vi "四点权值_黑子.vi"(0 "3位置行":dbl, 1 "2位置行":dbl, 2 "1位置行":dbl, 3 "当前棋盘状态":i32[][](array[numeric]), 5 "4位置行":dbl, 9 "1位置列":u8, 11 "2位置列":u8, 12 "3位置列":u8, 13 "4位置列":u8) -> (4 "黑子四位置权值":i32, 6 "有2个黑子?或黑子加无子?":bool, 8 "第1个位置是黑子?":bool, 10 "3个黑子?":bool, 14 "第一个位置为空":bool, 15 "3个黑子？或2个黑子加无子?":bool)   [LabVIEW 2018]
doc: "计算当前位置周围4个点的权值。"
panel:
  out "第四位在框内？":bool
  out "第三位在框内？":bool
  out "第二位在框内？":bool
  out "第一位在框内？":bool
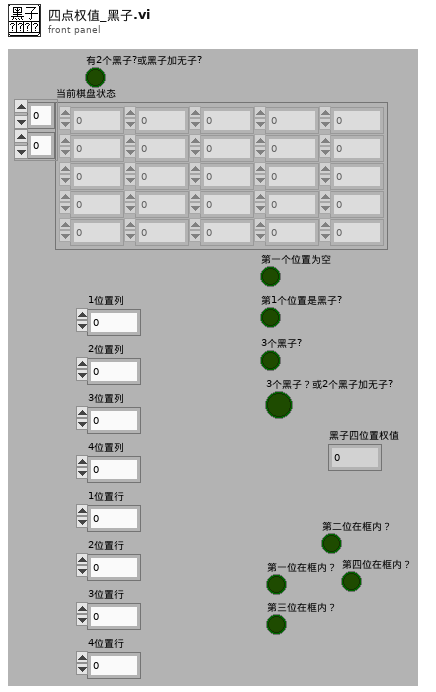
[diagram p1: front panel]
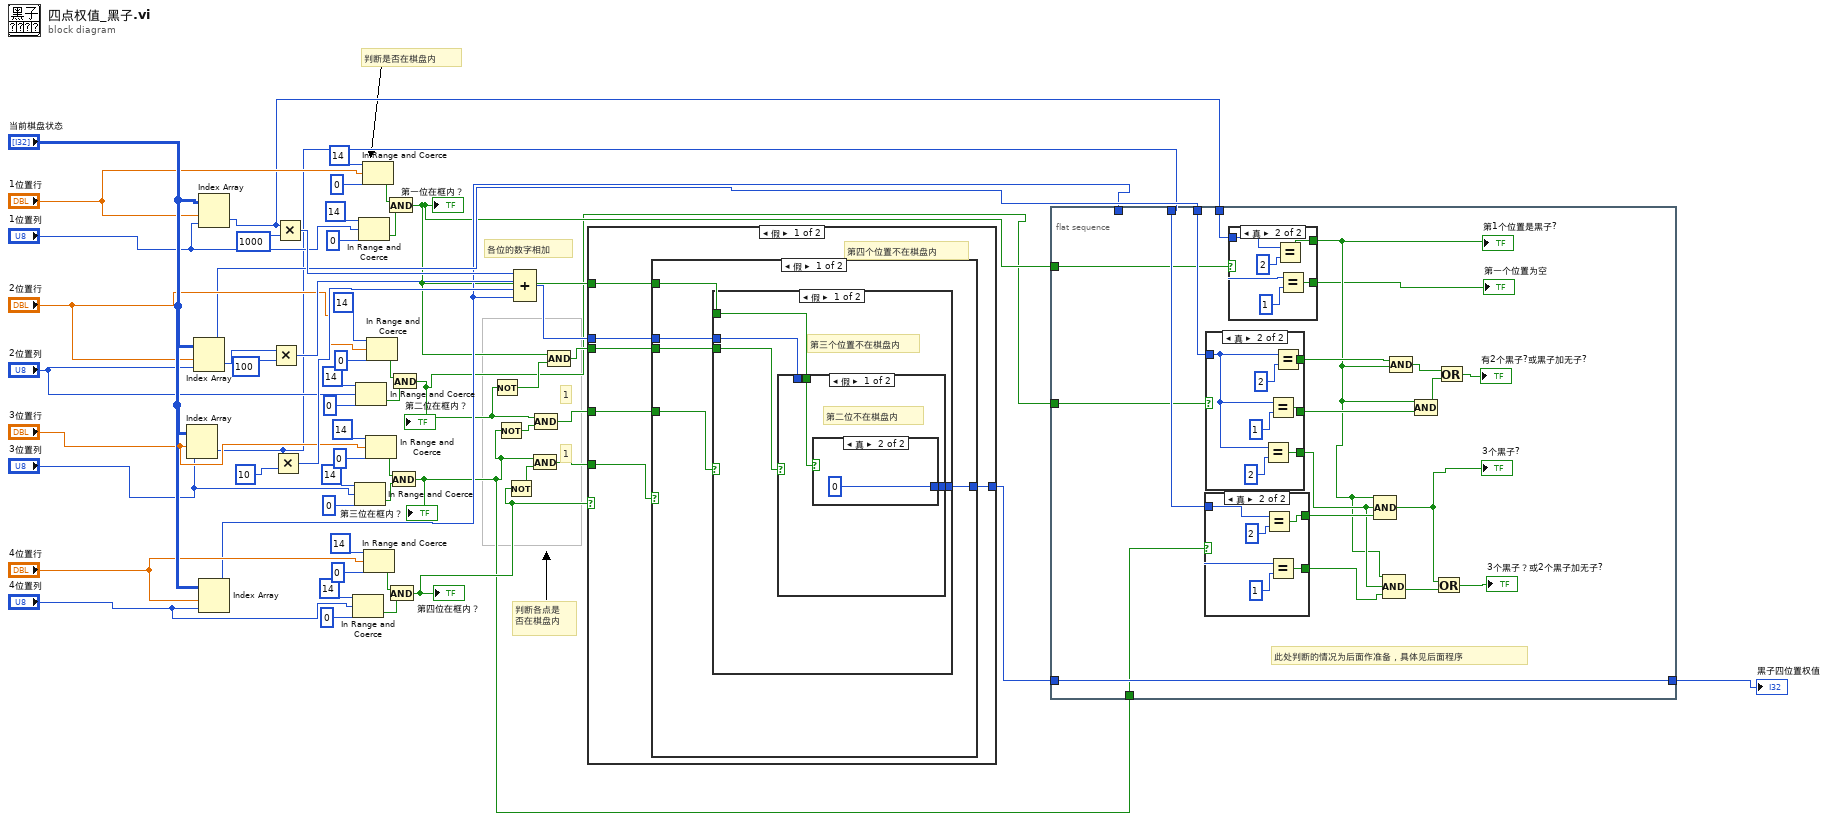
[diagram p0: block diagram]
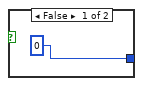
[diagram p2: hidden frame]
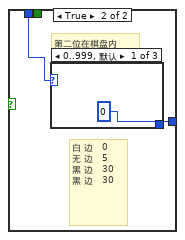
[diagram p3: hidden frame]
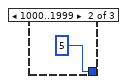
[diagram p4: hidden frame]
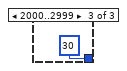
[diagram p5: hidden frame]
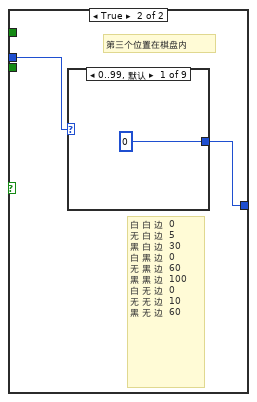
[diagram p6: hidden frame]
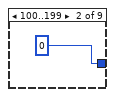
[diagram p7: hidden frame]
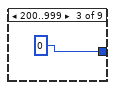
[diagram p8: hidden frame]
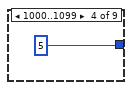
[diagram p9: hidden frame]
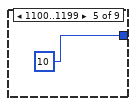
[diagram p10: hidden frame]
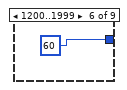
[diagram p11: hidden frame]
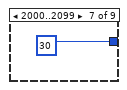
[diagram p12: hidden frame]
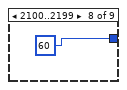
[diagram p13: hidden frame]
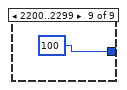
[diagram p14: hidden frame]
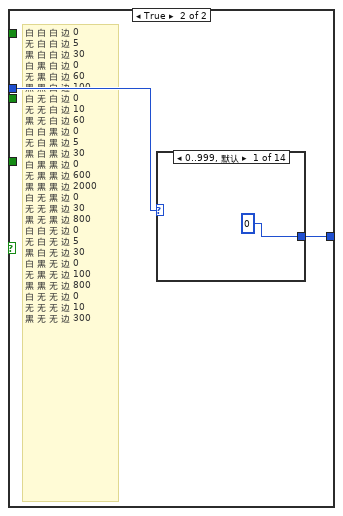
[diagram p15: hidden frame]
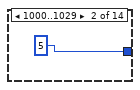
[diagram p16: hidden frame]
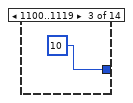
[diagram p17: hidden frame]
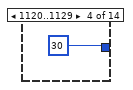
[diagram p18: hidden frame]
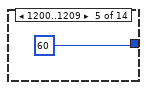
[diagram p19: hidden frame]
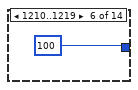
[diagram p20: hidden frame]
diagram:
  # "判断各点是\n否在棋盘内"
  # "各位的数字相加"
  # "判断是否在棋盘内"
  # "1"
  # "1"
  n1 = Index Array(array="当前棋盘状态", index (row)="3位置行", index (col)="3位置列") -> (element=w5:i32)
  n2 = Index Array(array="当前棋盘状态", index (row)="2位置行", index (col)="2位置列") -> (element=w6:i32)
  n3 = Index Array(array="当前棋盘状态", index (row)="1位置行", index (col)="1位置列") -> (element=w7:i32)
  n4 = Index Array(array="当前棋盘状态", index (row)="4位置行", index (col)="4位置列") -> (element=w4:i32)
  n5 = Multiply(x=w6, y=100) -> (x*y=w21:i32)
  n6 = Multiply(x=w5, y=10) -> (x*y=w20:i32)
  n7 = Multiply(x=w7, y=1000) -> (x*y=w22:i32)
  n8 = In Range and Coerce(upper limit=14, x="4位置列", lower limit=0) -> (In Range?=w36:bool)  [unwired: 1 out]
  n9 = In Range and Coerce(upper limit=14, x="3位置列", lower limit=0) -> (In Range?=w30:bool)  [unwired: 1 out]
  n10 = In Range and Coerce(upper limit=14, x="2位置列", lower limit=0) -> (In Range?=w50:bool)  [unwired: 1 out]
  n11 = In Range and Coerce(upper limit=14, x="1位置列", lower limit=0) -> (In Range?=w51:bool)  [unwired: 1 out]
  n12 = In Range and Coerce(upper limit=14, x="1位置行", lower limit=0) -> (In Range?=w52:bool)  [unwired: 1 out]
  n13 = In Range and Coerce(upper limit=14, x="4位置行", lower limit=0) -> (In Range?=w37:bool)  [unwired: 1 out]
  n14 = In Range and Coerce(upper limit=14, x="3位置行", lower limit=0) -> (In Range?=w31:bool)  [unwired: 1 out]
  n15 = In Range and Coerce(upper limit=14, x="2位置行", lower limit=0) -> (In Range?=w49:bool)  [unwired: 1 out]
  n16 = And(x=w52, y=w51) -> (x .and. y?=w3:bool)
  "第一位在框内？" <- w3
  n17 = And(x=w37, y=w36) -> (x .and. y?=w28:bool)
  "第四位在框内？" <- w28
  n18 = And(x=w31, y=w30) -> (x .and. y?=w1:bool)
  "第三位在框内？" <- w1
  n19 = And(x=w49, y=w50) -> (x .and. y?=w2:bool)
  "第二位在框内？" <- w2
  n20 = Not(x=w2) -> (.not. x?=w26:bool)
  n21 = Not(x=w1) -> (.not. x?=w24:bool)
  n22 = Not(x=w28) -> (.not. x?=w25:bool)
  n23 = Compound Arithmetic op=ADD(w22, w21, w20, w4) -> (w19:i32)
  n24 = And(x=w1, y=w25) -> (x .and. y?=w29:bool)
  n25 = Compound Arithmetic op=AND(w2, w24) -> (w27:bool)
  n26 = Compound Arithmetic op=AND(w3, w26) -> (w23:bool)
  n27 = case shown="假" w28 {
    tunnel: [w58 w109] -> w8
    tunnel: w29 -> [w62 _]
    tunnel: w27 -> [w61 _]
    tunnel: w23 -> [w60 _]
    tunnel: w3 -> [w59 _]
    tunnel: w19 -> [w57 w108]
    frame False {
      # "第四个位置不在棋盘内"
      n28 = case shown="假" w62 {
        tunnel: w61 -> [w67 _]
        tunnel: w60 -> [w66 _]
        tunnel: w59 -> [w65 _]
        tunnel: [w64 w92] -> w58
        tunnel: w57 -> [w63 w93]
        frame False {
          n29 = case shown="假" w67 {
            tunnel: w66 -> [w71 _]
            tunnel: w65 -> [w70 _]
            tunnel: [w69 w81] -> w64
            tunnel: w63 -> [w68 w82]
            frame False {
              # "第三个位置不在棋盘内"
              n30 = case shown="假" w71 {
                tunnel: w70 -> [w73 _]
                tunnel: [w72 w76] -> w69
                tunnel: w68 -> [_ w77]
                frame False {
                  # "第二位不在棋盘内"
                  n31 = case shown="真" w73 {
                    tunnel: [0 0] -> w72
                    frame False {
                    }
                    frame True {
                    }
                  }
                }
                frame True {
                  # "第二位在棋盘内"
                  # "白\t边\t\t\t0\n无\t边\t\t\t5\n黑\t边\t\t\t30\n黑\t边\t\t\t30"
                  n32 = case shown="0..999, 默认" w77 {
                    tunnel: [0 5 30] -> w76
                    frame 0..999, Default {
                    }
                    frame 1000..1999 {
                    }
                    frame 2000..2999 {
                    }
                  }
                }
              }
            }
            frame True {
              # "第三个位置在棋盘内"
              # "白\t白\t边\t\t0\n无\t白\t边\t\t5\n黑\t白\t边\t\t30\n白\t黑\t边\t\t0\n无\t黑\t边\t\t60\n黑\t黑\t边\t\t100\n白\t无\t边\t\t0\n无\t无\t边\t\t10\n黑\t无\t边\t\t60"
              n33 = case shown="0..99, 默认" w82 {
                tunnel: [0 0 0 5 10 60 30 60 100] -> w81
                frame 0..99, Default {
                }
                frame 100..199 {
                }
                frame 200..999 {
                }
                frame 1000..1099 {
                }
                frame 1100..1199 {
                }
                frame 1200..1999 {
                }
                frame 2000..2099 {
                }
                frame 2100..2199 {
                }
                frame 2200..2299 {
                }
              }
            }
          }
        }
        frame True {
          # "白\t白\t白\t边\t0\n无\t白\t白\t边\t5\n黑\t白\t白\t边\t30\n白\t黑\t白\t边\t0\n无\t黑\t白\t边\t60\n黑\t黑\t白\t边\t100\n白\t无\t白\t边\t0\n无\t无\t白\t边\t10\n黑\t无\t白\t边\t60\n白\t白\t黑\t边\t0\n无\t白\t黑\t边\t5\n黑\t白\t黑\t边\t30\n白\t黑\t黑\t边\t0\n无\t黑\t黑\t边\t600\n黑\t黑\t黑\t边\t2000\n白\t无\t黑\t边\t0\n无\t无\t黑\t边\t30\n黑\t无\t黑\t边\t800\n白\t白\t无\t边\t0\n无\t白\t无\t边\t5\n黑\t白\t无\t边\t30\n白\t黑\t无\t边\t0\n无\t黑\t无\t边\t100\n黑\t黑\t无\t边\t800\n白\t无\t无\t边\t0\n无\t无\t无\t边\t10\n黑\t无\t无\t边\t300"
          n34 = case shown="0..999, 默认" w93 {
            tunnel: [0 5 10 30 60 100 600 30 60 300 800 100 800 2000] -> w92
            frame 0..999, Default {
            }
            frame 1000..1029 {
            }
            frame 1100..1119 {
            }
            frame 1120..1129 {
            }
            frame 1200..1209 {
            }
            frame 1210..1219 {
            }
            frame 1220..1229 {
            }
            frame 2000..2029 {
            }
            frame 2100..2109 {
            }
            frame 2110..2119 {
            }
            frame 2120..2129 {
            }
            frame 2200..2209 {
            }
            frame 2210..2219 {
            }
            frame 2220 {
            }
          }
        }
      }
    }
    frame True {
      # "第四个仍在棋盘内"
      # "无\t黑\t黑\t白\t600\n黑\t黑\t黑\t白\t2000\n无\t无\t黑\t白\t30\n黑\t无\t黑\t白\t800\n无\t黑\t无\t白\t100\n黑\t黑\t无\t白\t800\n无\t无\t无\t白\t10\n黑\t无\t无\t白\t300"
      # "无\t黑\t黑\t黑\t50000\n黑\t黑\t黑\t黑\t1000000\n无\t无\t黑\t黑\t2000\n黑\t无\t黑\t黑\t50000\n无\t黑\t无\t黑\t2000\n黑\t黑\t无\t黑\t50000\n无\t无\t无\t黑\t400\n黑\t无\t无\t黑\t2000\n无\t黑\t黑\t无\t5000\n黑\t黑\t黑\t无\t100000\n无\t无\t黑\t无\t600\n黑\t无\t黑\t无\t5000\n无\t黑\t无\t无\t8000\n黑\t黑\t无\t无\t10000\n无\t无\t无\t无\t100\n黑\t无\t无\t无\t1000"
      n35 = case shown="2122" w108 {
        tunnel: [5 5 10 100 400 10 30 600 2000 30 10 60 100 800 2000 100 600 5000 5000 600 60 5 30 60 300 1000 2000 300 800 5000 50000 800 60 100 800 10000 50000 800 2000 100000 1000000 2000 100 30 0 0] -> w109
        frame 1000..1099 {
        }
        frame 1100..1109 {
        }
        frame 1110 {
        }
        frame 1111 {
        }
        frame 1112 {
        }
        frame 1113 {
        }
        frame 1120 {
        }
        frame 1121 {
        }
        frame 1122 {
        }
        frame 1123 {
        }
        frame 1130..1139 {
        }
        frame 1200..1209 {
        }
        frame 1210 {
        }
        frame 1211 {
        }
        frame 1212 {
        }
        frame 1213 {
        }
        frame 1220 {
        }
        frame 1221 {
        }
        frame 1222 {
        }
        frame 1223 {
        }
        frame 1230..1239 {
        }
        frame 1300..1399 {
        }
        frame 2000..2099 {
        }
        frame 2100..2109 {
        }
        frame 2110 {
        }
        frame 2111 {
        }
        frame 2112 {
        }
        frame 2113 {
        }
        frame 2120 {
        }
        frame 2121 {
        }
        frame 2122 {
        }
        frame 2123 {
        }
        frame 2130..2139 {
        }
        frame 2200..2209 {
        }
        frame 2210 {
        }
        frame 2211 {
        }
        frame 2212 {
        }
        frame 2213 {
        }
        frame 2220 {
        }
        frame 2221 {
        }
        frame 2222 {
        }
        frame 2223 {
        }
        frame 2230..2239 {
        }
        frame 2300..2399 {
        }
        frame 3000..3999 {
        }
        frame 0..999, Default {
        }
      }
    }
  }
  n36 = flat-sequence {
    tunnel: [w162] -> w9
    tunnel: w8 -> [w162]
    tunnel: w7 -> [w161]
    tunnel: w6 -> [w160]
    tunnel: w5 -> [w159]
    tunnel: w4 -> [_]
    tunnel: w3 -> [w158]
    tunnel: w2 -> [w157]
    tunnel: w1 -> [w156]
    frame #0 {
      # "此处判断的情况为后面作准备，具体见后面程序"
      n37 = case shown="真" w156 {
        tunnel: [w176 w180] -> w175
        tunnel: [w176 w178] -> w165
        tunnel: w159 -> [_ w177]
        frame False {
          w176 = FALSE
        }
        frame True {
          n38 = Equal?(x=w177, y=2) -> (x = y?=w180:bool)
          n39 = Equal?(x=w177, y=1) -> (x = y?=w178:bool)
        }
      }
      n40 = case shown="真" w157 {
        tunnel: [w182 w187] -> w174
        tunnel: [w182 w185] -> w172
        tunnel: [w182 w184] -> w169
        tunnel: w160 -> [_ w183]
        frame False {
          w182 = FALSE
        }
        frame True {
          n41 = Equal?(x=w183, y=2) -> (x = y?=w184:bool)
          n42 = Equal?(x=w183, y=1) -> (x = y?=w187:bool)
          n43 = Equal?(x=w183, y=2) -> (x = y?=w185:bool)
        }
      }
      n44 = case shown="真" w158 {
        tunnel: [w190 w194] -> w168
        tunnel: [w190 w192] -> w164
        tunnel: w161 -> [_ w191]
        frame False {
          w190 = FALSE
        }
        frame True {
          n45 = Equal?(x=w191, y=2) -> (x = y?=w194:bool)
          n46 = Equal?(x=w191, y=1) -> (x = y?=w192:bool)
        }
      }
      "第1个位置是黑子?" <- w168
      "第一个位置为空" <- w164
      n47 = Compound Arithmetic op=AND(w168, w169, w175) -> (w163:bool)
      "3个黑子?" <- w163
      n48 = Compound Arithmetic op=AND(w168, w169, w165) -> (w167:bool)
      n49 = Compound Arithmetic op=AND(w172, w168) -> (w171:bool)
      n50 = Compound Arithmetic op=AND(w168, w174) -> (w173:bool)
      n51 = Or(x=w163, y=w167) -> (x .or. y?=→"3个黑子？或2个黑子加无子?":bool)
      n52 = Or(x=w171, y=w173) -> (x .or. y?=→"有2个黑子?或黑子加无子?":bool)
    }
  }
  "黑子四位置权值" <- w9
